vi "v0.2_Rotar_Angulo_http.vi"(4 "PA:13":u32=1, 6 "PA:12":u32=1, 8 "error in":errorcluster, 9 "Vel. Rotacion":u32=10000, 10 "Angulo":dbl, 11 "mbed.lvclass IN":refnum<class "mbed.lvclass">) -> (0 "error out":errorcluster, 3 "mbed.lvclass OUT":refnum<class "mbed.lvclass">)   [LabVIEW 2011]
uses:
  C:/mbed/Transport Mechanisms/mbed/mbed.lvclass
panel:
  # "Rotar Ángulo"
  # "Posicionamiento relativo, no absoluto, \nes decir, incrementa o decrementa el \nángulo a partir de la posición actual del\nmotor"
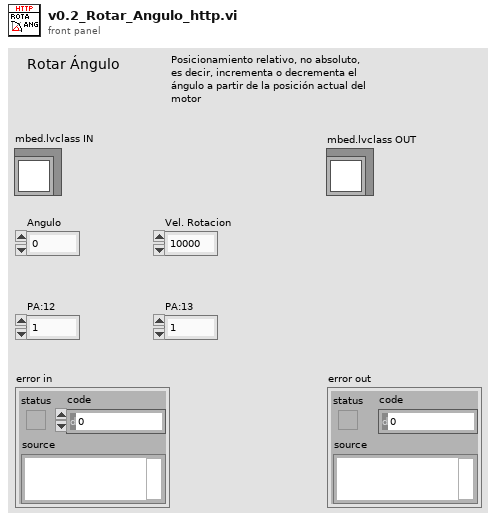
[diagram p1: front panel]
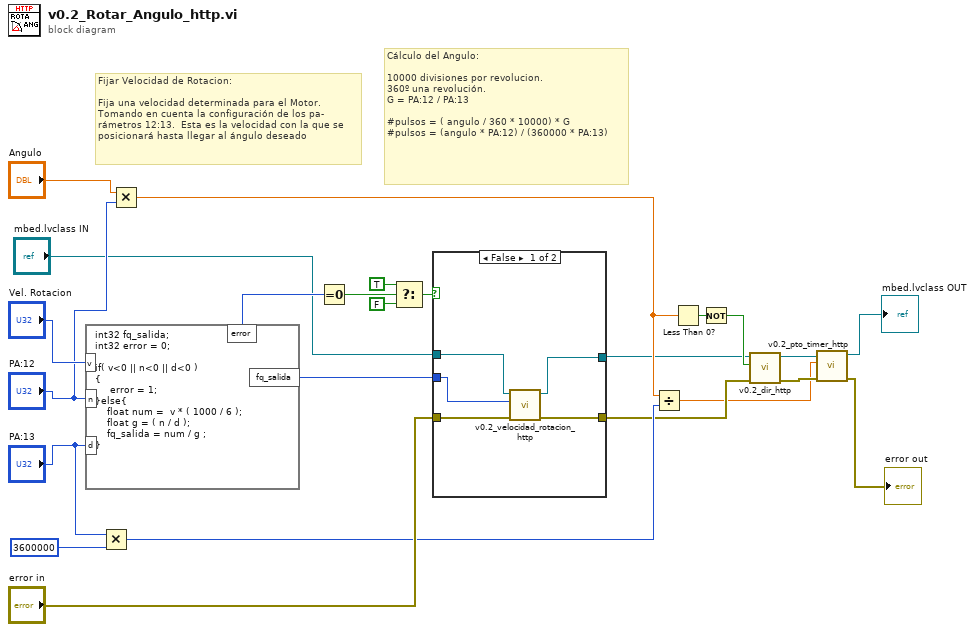
[diagram p0: block diagram]
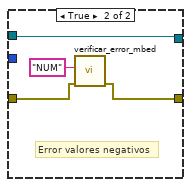
[diagram p2: hidden frame]
diagram:
  # "Cálculo del Angulo:\n\n10000 divisiones por revolucion.\n360º una revolución.\nG = PA:12 / PA:13\n\n#pulsos = ( angulo / 360 * 10000) * G\n#pulsos = (angulo * PA:12) / (360000 * PA:13)"
  # "Fijar Velocidad de Rotacion:\n\nFija una velocidad determinada para el Motor.  \nTomando en cuenta la configuración de los pa-\nrámetros 12:13.  Esta es la velocidad con la que se \nposicionará hasta llegar al ángulo deseado"
  n1 = formula code="int32 fq_salida;\nint32 error = 0;\n\nif( v<0 || n<0 || d<0 )\n{\n     error = 1; \n}else{\n    float num =  v * ( 1000 / 6 );\n    float g = ( n / d );\n    fq_salida = num / g ;\n}"("v"="Vel. Rotacion", "n"="PA:12", "d"="PA:13") -> ("fq_salida"=w24:i32, "error"=w23:i32)
  n2 = Multiply(x="PA:13", y=3600000) -> (x*y=w11:u32)
  n3 = Multiply(x="Angulo", y="PA:12") -> (x*y=w10:dbl)
  n4 = Equal To 0?(x=w23) -> (x = 0?=w22:bool)
  n5 = Select(t=TRUE, s=w22, f=FALSE) -> (s? t:f=w19:bool)
  n6 = case shown="False" w19 {
    tunnel: w24 -> [w28 _]
    tunnel: "error in" -> [w27 w32]
    tunnel: [w26 w31] -> w7
    tunnel: "mbed.lvclass IN" -> [w29 w33]
    tunnel: [w25 w33] -> w2
    frame False {
      n7 = call "v0.2_velocidad_rotacion_http.vi"("error in"=w27, "Freq Rotacion"=w28, "mbed.lvclass IN"=w29) -> ("error out"=w26:errorcluster, "mbed.lvclass OUT"=w25:refnum<class "mbed.lvclass">)  [unwired: 7 in]
    }
    frame True {
      # "Error valores negativos"
      n8 = call "verificar_error_mbed.vi"("error in (no error)"=w32, "desde_mbed"="NUM") -> ("error out"=w31:errorcluster)  [unwired: 8 in, 1 out]
    }
  }
  n9 = Divide(x=w10, y=w11) -> (x/y=w4:dbl)
  n10 = Less Than 0?(x=w10) -> (x < 0?=w9:bool)
  n11 = Not(x=w9) -> (.not. x?=w8:bool)
  n12 = call "v0.2_dir_http.vi"("error in (no error)"=w7, "Direccion"=w8, "mbed.lvclass IN"=w2) -> ("error out"=w5:errorcluster, "mbed.lvclass OUT"=w6:refnum<class "mbed.lvclass">)  [unwired: 7 in]
  n13 = call "v0.2_pto_timer_http.vi"("error in"=w5, "n pulsos"=w4, "mbed.lvclass IN"=w6) -> ("error out"=→"error out":errorcluster, "mbed.lvclass OUT"=→"mbed.lvclass OUT":refnum<class "mbed.lvclass">)  [unwired: 7 in]
